vi "State data Look up string key.vi"(6 "Error on not found (T)":bool=TRUE, 7 "Key [string/enum]":variant, 8 "error in (no error)":errorcluster, 10 "Value if not found (\"\")":string, 11 "Fiber Auto Collimation state data in":refnum<class "Fiber Auto Collimation state data.lvclass">) -> (0 "error out":errorcluster, 1 "String Key found":bool, 2 "String Key Value":string, 3 "Fiber Auto Collimation state data out":refnum<class "Fiber Auto Collimation state data.lvclass">)   [LabVIEW 2018, in "Fiber Auto Collimation state data.lvclass"]
doc: "Serial number of the Device Under Test."
uses:
  Fiber Auto Collimation state data.lvclass
  Fiber Auto Collimation state data.lvclass/Fiber Auto Collimation state data.ctl
  <userlib>/Recipe/Test Recipe classes/Test Recipe.lvclass
  C:/Program Files (x86)/National Instruments/LabVIEW 2018/user.lib/Recipe/nLight Recipe/nLight Recipe.lvclass
  <userlib>/Recipe/nLight Recipe/nLight Recipe.lvclass
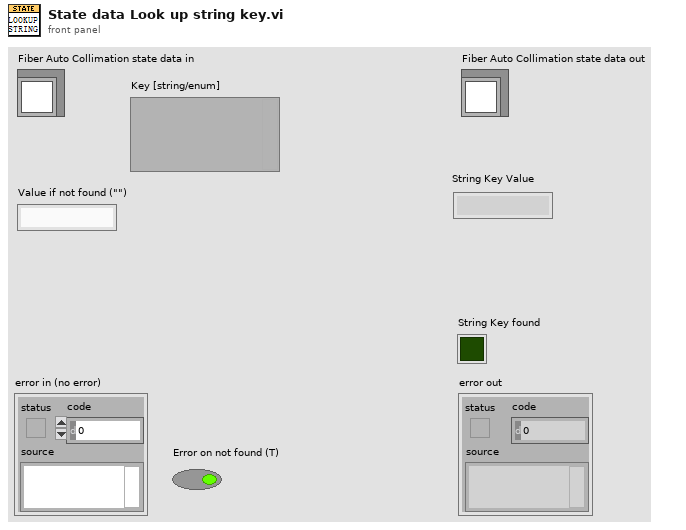
[diagram p1: front panel]
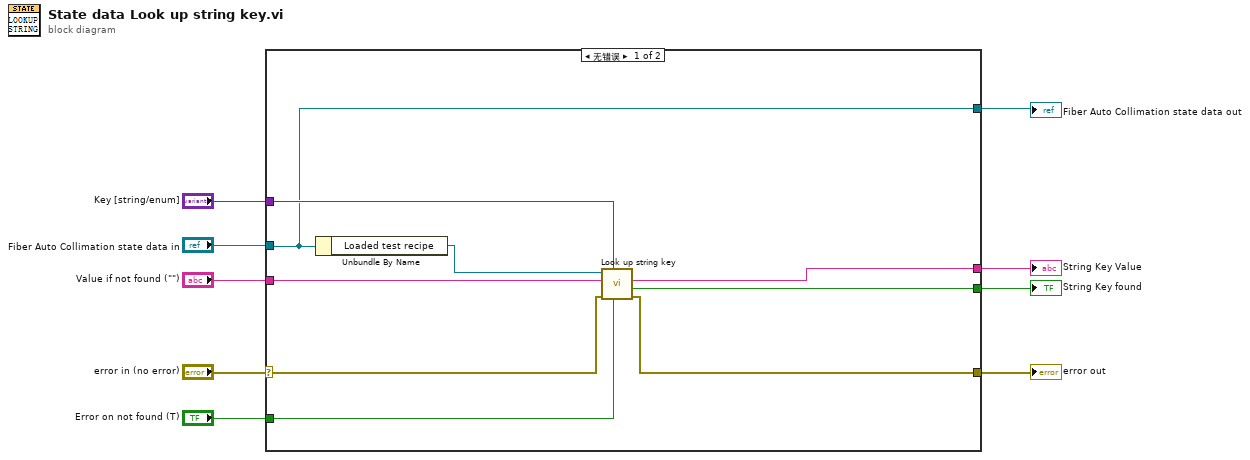
[diagram p0: block diagram]
diagram:
  n1 = case shown="无错误" "error in (no error)" {
    selector: "error in (no error)" -> [w16 w20]
    tunnel: [w13 w20] -> w8
    tunnel: [w14 w19] -> w3
    tunnel: "Fiber Auto Collimation state data in" -> [w14 w19]
    tunnel: "Key [string/enum]" -> [w15 _]
    tunnel: "Error on not found (T)" -> [w12 _]
    tunnel: [w10 _] -> w1
    tunnel: [w11 _] -> w5
    tunnel: "Value if not found (\"\")" -> [w18 _]
    frame No Error {
      n2 = Unbundle By Name(w14) -> ("Loaded test recipe"=w17:refnum<class "Test Recipe.lvclass">)
      n3 = call <userlib>:"Look up string key.vi"("Error on not found (T)"=w12, "Key [string/enum]"=w15, "error in (no error)"=w16, "Value if not found (\"\")"=w18, "nLight Recipe in"=w17) -> ("error out"=w13:errorcluster, "String Key found"=w11:bool, "String Key Value"=w10:string)  [unwired: 3 in, 1 out]
    }
    frame Error {
    }
  }
  "Fiber Auto Collimation state data out" <- w3
  "error out" <- w8
  "String Key found" <- w5
  "String Key Value" <- w1
